vi "Set parameter.vi"(3 "霍尔参数":u16[](array[numeric])) -> (0 "设定":bool, 1 "输出参数":u16[](array[numeric]))   [LabVIEW 2018]
panel:
  in  "取消":bool
  in  "确定":bool
  in  "全关位置":u16
  in  "全开位置":u16
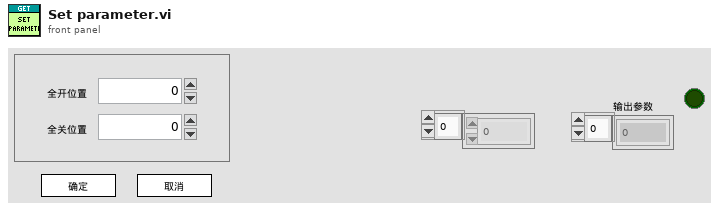
[diagram p1: front panel]
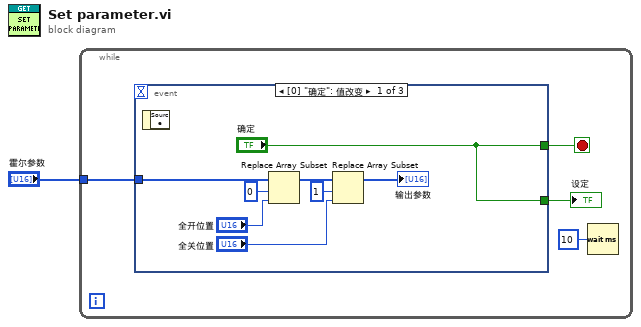
[diagram p0: block diagram]
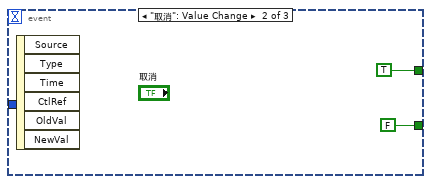
[diagram p2: hidden frame]
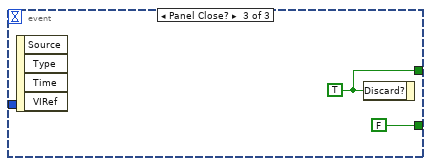
[diagram p3: hidden frame]
diagram:
  n1 = while {
    tunnel: "霍尔参数" -> [w5]
    stop <- w4 stop-if-true
    n2 = event shown="[0] \"确定\": 值改变" {
      selector: _ -> [_ _ _]
      dyn-events: _ -> [_ _ _]
      timeout: _ -> [_ _ _]
      tunnel: ["确定" TRUE ("确定") w17] -> w4
      tunnel: w5 -> [w12 _ _]
      tunnel: ["确定" FALSE ("确定") FALSE ("确定")] -> w3
      event "确定": Value Change {
        n3 = event-data() -> ()  [unwired: 1 in, 1 out]
        n4 = Replace Array Subset(array=w12, new element="全开位置", index=0 ("索引")) -> (w9:u16[])
        n5 = Replace Array Subset(array=w9, new element="全关位置", index=1 ("索引")) -> (→"输出参数":u16[])
      }
      event "取消": Value Change {
        n6 = event-data() -> ()  [unwired: 1 in, 6 out]
      }
      event Panel Close? {
        w17 = TRUE ("放弃？")
        n7 = event-data() -> ()  [unwired: 1 in, 4 out]
        n8 = event-data("Discard?"=w17) -> ()  [unwired: 1 in, 1 out]
      }
    }
    "设定" <- w3
    n9 = Wait (ms)(milliseconds to wait=u32 10 ("等待时间（毫秒）")) -> ()  [unwired: 1 out]
  }
